vi "Set Duty Cycle N Chans.vi"(8 "Error In":errorcluster, 9 "Duty Cycles":u8[](array[numeric]), 10 "PWM Channels":u8[](array[numeric]), 11 "LINX Resource":T1) -> (0 "Error Out":errorcluster, 3 "LINX Resource":T1)   [LabVIEW 2011, in "LVH-LINX.lvlib"]
doc: "Set the duty cycle of the specified PWM channels. \n\nA duty cycle of 0 coresponds to 0% on and a duty cycle of 255 coresponds to 100% on."
uses:
  LVH-LINX.lvlib
  Private/Type Defs/LINX Ref.ctl
  Private/Type Defs/Platform.ctl
  Private/Type Defs/Interface.ctl
  Private/Device/Type Defs/LINX Device Config.ctl
  Private/Device/Type Defs/TCP Config.ctl
  Private/Device/Type Defs/Channels.ctl
  Private/Type Defs/Peripheral.ctl
  Private/Device/Device.lvlib
  Private/myRIO/myRIO.lvlib
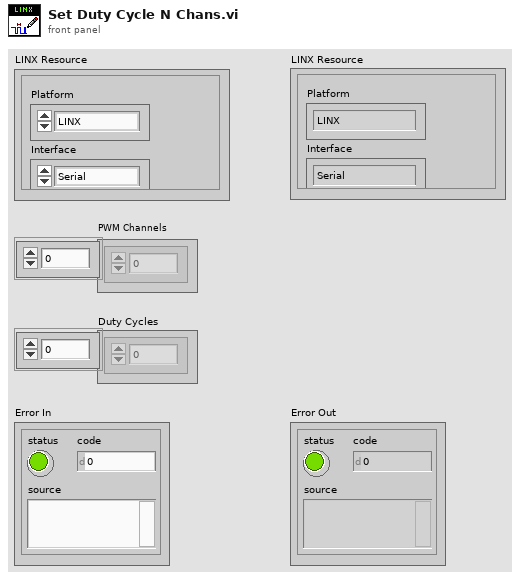
[diagram p1: front panel]
types:
  T1 = typedef "LVH-LINX.lvlib/LINX Ref.ctl" = cluster{"Platform":T2, "Interface":T3, "LINX Device Config":T4}
  T2 = typedef "LVH-LINX.lvlib/Platform.ctl" = enum16{"LINX", "myRIO"}
  T3 = typedef "LVH-LINX.lvlib/Interface.ctl" = enum16{"Serial", "TCP"}
  T4 = typedef "LVH-LINX.lvlib/Device.lvlib/LINX Device Config.ctl" = cluster{"Interface":T3, "COM Port":refnum<visa-resource-name>, "TCP Configuration":T5, "Device Family":u8, "Device ID":u8, "Device Name":string, "TCP Ref":refnum<k5>, "Channels":T6}
  T5 = typedef "LVH-LINX.lvlib/Device.lvlib/TCP Config.ctl" = cluster{"IP Address":string, "Port":u16}
  T6 = typedef "LVH-LINX.lvlib/Channels.ctl" = cluster{"DI":u8[], "DO":u8[], "AI":u8[], "AO":u8[], "PWM":u8[], "QE":u8[], "UART":u8[], "I2C 2":u8[], "SPI":u8[], "CAN":u8[], "Servo":u8[], "AI Ref (V)":dbl, "AO Ref (V)":dbl, "AO Resolution (Bits)":u8}
  T7 = typedef "LVH-LINX.lvlib/Peripheral.ctl" = enum8{"DI", "DO", "AI", "AO", "PWM", "QE", "UART", "I2C", "SPI", "CAN", "Servo"}
  T8 = typedef "PWM.lvlib/PWM Reference.ctl" = cluster{"myRIO Reference":T9, "PWM Channels Enum":T13, "PWM Configuration":T14}
  T9 = typedef "myRIO Generic Hardware Reference.ctl" = cluster{"myRIO Model":T10, "myRIO Hardware Reference":T11}
  T10 = typedef "Hardware Version Enum.ctl" = enum16{"Unknown", "myRIO-1900", "myRIO-1950"}
  T11 = typedef "myRIO v1.0 Reference.ctl" = cluster{"Generic FPGA Reference":T12, "Allow multiple opens":bool}
  T12 = typedef "Generic FPGA Reference.ctl" = refnum<k20>
  T13 = typedef "PWM Channels Enum.ctl" = enum16{"Not Connected", "C/PWM0", "C/PWM1", "A/PWM0", "A/PWM1", "A/PWM2", "B/PWM0", "B/PWM1", "B/PWM2"}
  T14 = typedef "PWM.lvlib/PWM Configuration.ctl" = cluster{"Frequency":dbl, "Duty Cycle":dbl}
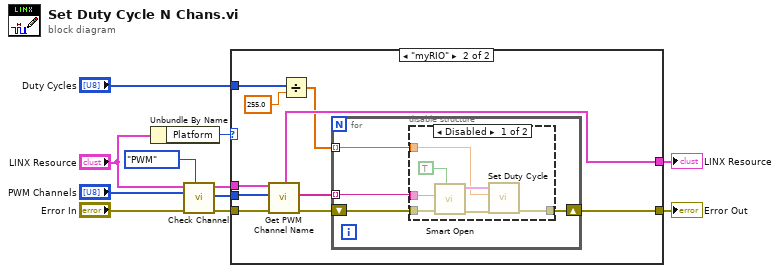
[diagram p0: block diagram]
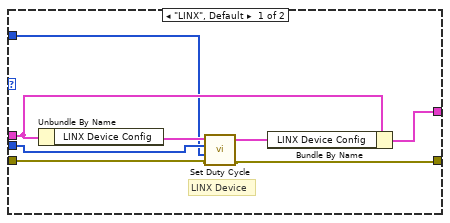
[diagram p2: hidden frame]
diagram:
  n1 = Unbundle By Name("LINX Resource") -> ("Platform"=w11:T2)
  n2 = call "Check Channel.vi"("Peripheral"=Peripheral."PWM", "Error In"="Error In", "Channels"="PWM Channels", "LINX Resource"="LINX Resource") -> ("Error Out"=w4:errorcluster, "Channels"=w3:u8[], "LINX Resource"=w6:T1)  [unwired: 5 in]
  n3 = case shown="\"myRIO\"" w11 {
    tunnel: w4 -> [w16 w27]
    tunnel: w6 -> [w19 w28]
    tunnel: [w17 w24] -> w10
    tunnel: [w18 w28] -> w9
    tunnel: "Duty Cycles" -> [w12 w22]
    tunnel: w3 -> [w13 w26]
    frame "LINX", Default {
      # "LINX Device"
      n4 = Unbundle By Name(w19) -> ("LINX Device Config"=w14:T4)
      n5 = call <vilib>:"Set Duty Cycle.vi"("Error In"=w16, "Duty Cycles (0-255)"=w12, "Channels"=w13, "LINX Device Config"=w14) -> ("Error Out"=w17:errorcluster, "LINX Device Config"=w15:T4)  [unwired: 6 in]
      n6 = Bundle By Name(cluster=w19, "LINX Device Config"=w15) -> (w18:T1)
    }
    frame "myRIO" {
      n7 = call "Get PWM Channel Name.vi"("Error In"=w27, "PWM Channel Nums"=w26) -> ("Error Out"=w25:errorcluster, "PWM Channels"=w23:string[])  [unwired: 8 in]
      n8 = Divide(x=w22, y=255.0) -> (x/y=w20:dbl[])
      n9 = for {
        shift-right: [w32] -> w24
        shift-left: w25 -> [w31]
        tunnel: w23 -> [w30] mode=indexing
        tunnel: w20 -> [w29] mode=indexing
        n10 = disable-structure shown="Disabled" {
          disable-tunnel: [w36 w40] -> w32
          disable-tunnel: w31 -> [w35 w40]
          disable-tunnel: w30 -> [w34 _]
          disable-tunnel: w29 -> [w33 _]
          frame Disabled {
            n11 = call <vilib>:"Smart Open.vi"("Allow multiple opens?"=TRUE, "error in (no error)"=w35, "Channel Name"=w34) -> ("error out"=w39:errorcluster, "PWM Ref Out"=w38:T8)  [unwired: 7 in]
            n12 = call <vilib>:"Set Duty Cycle.vi"("error in (no error)"=w39, "Duty Cycle (0-1)"=w33, "PWM Ref In"=w38) -> ("error out"=w36:errorcluster)  [unwired: 6 in, 1 out]
          }
          frame Enabled {
          }
        }
      }
    }
  }
  "Error Out" <- w10
  "LINX Resource" <- w9
